vi "Search 1D String Array 2012 NIVerified.vi"() -> ()   [LabVIEW 2018]
doc: "This VI makes use of the search/split string function to find matches of a search term in a string array. For example, if you have an array with the following elements:\nElement1\nElement2\nElement3\nVariable1\nVariable2\nVariable3\nYou could search for Element to return an array of both the results Element1, Element2, Element 3 and their indices 0, 1 and 2.\nThe Input Array and Search Term terminals accept a 1d array of strings and an individual string respectively.\nThe Match Indices and Match Values outputs return 1d arrays of long integers and strings respectively."
panel:
  out "Matches?":bool
  in  "Search Term":string
  in  "Input Array":string[](array[string])
  out "Match Values":string[](array[string])
  out "Match Indices":i32[](array[numeric])
  # "Overview: This VI is for finding and returning matches to a search string within a 1d string array and the respective indices of the results.\nRequirements: LabVIEW 2012 (or compatible)\nInstructions:\n1. Input the search term to be searched in the input array.\n2. Input the string array.\n3. Run VI.\n4. Match Indices and Match Values show the result corresponding to each element of the Input array."
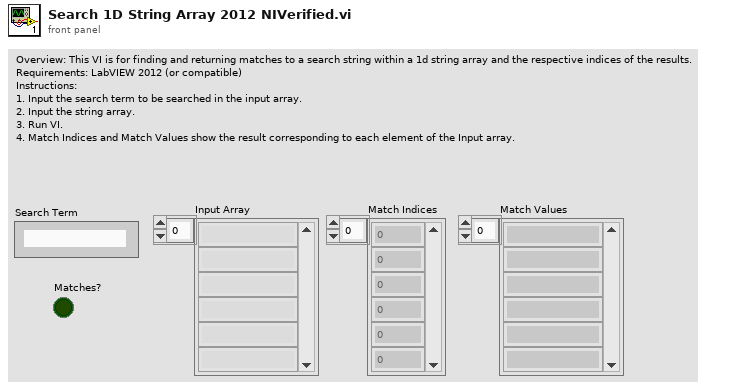
[diagram p1: front panel]
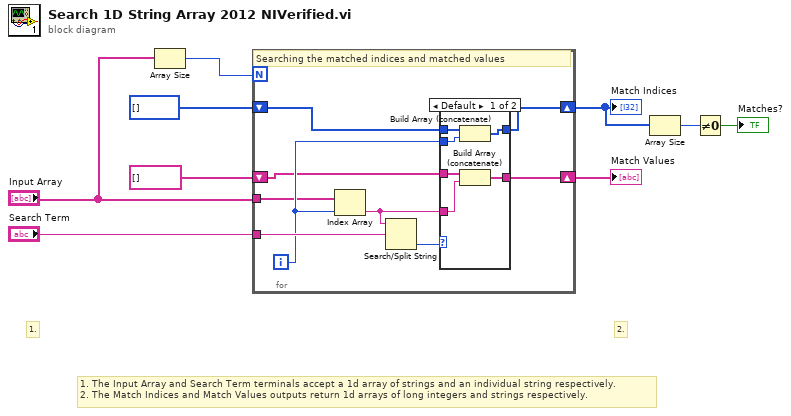
[diagram p0: block diagram]
diagram:
  # "2."
  # "1."
  # "1. The Input Array and Search Term terminals accept a 1d array of strings and an individual string respectively.\n2. The Match Indices and Match Values outputs return 1d arrays of long integers and strings respectively."
  n1 = Array Size(array="Input Array") -> (size(s)=w6:i32)
  n2 = for {
    N: w6 -> [_]
    tunnel: "Input Array" -> [w11]
    tunnel: "Search Term" -> [w16]
    shift-right: [w17] -> w4
    shift-left: i32[] [] ("in2") -> [w18]
    shift-right: [w12] -> w9
    shift-left: string[] [] -> [w10]
    i -> [w13]
    # "Searching the matched indices and matched values"
    n3 = Index Array(array=w11, index=w13) -> (element=w14:string)
    n4 = Search/Split String(string=w14, search string/char (-)=w16) -> (offset of match=w15:i32)  [unwired: 1 in, 2 out]
    n5 = case shown="Default" w15 {
      tunnel: [w19 w25] -> w12
      tunnel: w13 -> [w24 _]
      tunnel: [w23 w26] -> w17
      tunnel: w18 -> [w22 w26]
      tunnel: w14 -> [w20 _]
      tunnel: w10 -> [w21 w25]
      frame Default {
        n6 = Build Array (concatenate)(w22, w24) -> (w23:i32[])
        n7 = Build Array (concatenate)(w21, w20) -> (w19:string[])
      }
      frame -1 {
      }
    }
  }
  "Match Indices" <- w4
  "Match Values" <- w9
  n8 = Array Size(array=w4) -> (size(s)=w3:i32)
  n9 = Not Equal To 0?(x=w3) -> (x != 0?=→"Matches?":bool)
